vi "BuildConstructor.vi"(7 "PythonConverter_BD in":refnum<class "PyConvBD.lvclass">, 8 "error in":errorcluster, 11 "SubVI in":refnum<class "SubVI.lvclass">) -> (0 "error out":errorcluster, 3 "SubVI out":refnum<class "SubVI.lvclass">, 4 "constructor":string, 5 "PythonConverter_BD out":refnum<class "PyConvBD.lvclass">)   [LabVIEW 2014, in "Raspberry Pi Compatible Compiler for LabVIEW.lvlib" / "SubVI.lvclass"]
uses:
  SubVI.lvclass
  Python/PythonConverter_BD/PyConvBD.lvclass
  SubVI.lvclass/SubVI.ctl
  Node/Node.lvclass
  Python/Parsing/Python Functions.lvlib
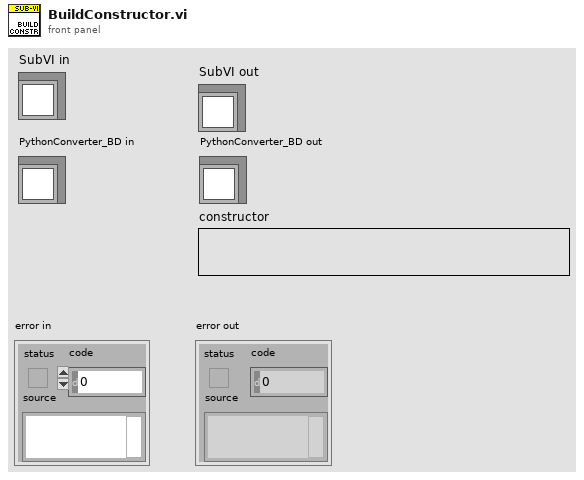
[diagram p1: front panel]
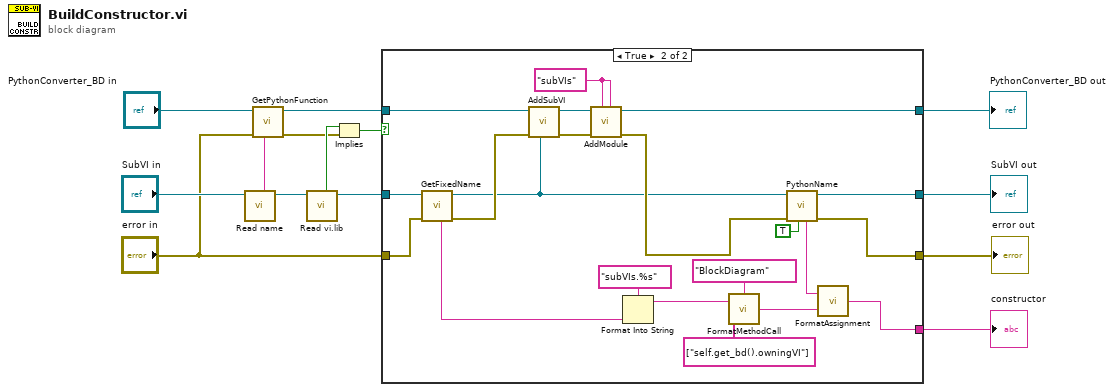
[diagram p0: block diagram]
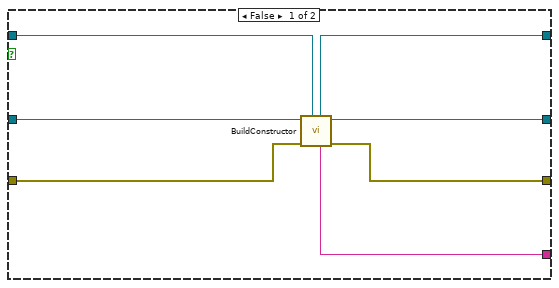
[diagram p2: hidden frame]
diagram:
  n1 = call-dynamic "Read name.vi"("SubVI in"="SubVI in") -> ("SubVI out"=w5:refnum<class "SubVI.lvclass">, "name"=w8:string)  [unwired: 7 in]
  n2 = call "GetPythonFunction.vi"("function name"=w8, "error in"="error in", "PythonConverter_BD in"="PythonConverter_BD in") -> ("error out"=w2:errorcluster, "PythonConverter_BD out"=w9:refnum<class "PyConvBD.lvclass">)  [unwired: 4 in, 1 out]
  n3 = call "Read vi.lib.vi"("SubVI in"=w5) -> ("SubVI out"=w4:refnum<class "SubVI.lvclass">, "vi.lib"=w6:bool)  [unwired: 7 in]
  n4 = Implies(1:w2, 2:w6) -> (0:w7:bool)
  n5 = case shown="True" w7 {
    tunnel: [w15 w37] -> w14
    tunnel: [w21 w38] -> w13
    tunnel: [w20 w34] -> w12
    tunnel: [w19 w32] -> w11
    tunnel: w9 -> [w18 w26]
    tunnel: w4 -> [w17 w29]
    tunnel: "error in" -> [w16 w28]
    frame False {
      n6 = call-parent "BuildConstructor.vi"("PythonConverter_BD in"=w18, "error in"=w16, "Node in"=w17) -> ("error out"=w15:errorcluster, "Node out"=w21:refnum<class "SubVI.lvclass">, "constructor"=w20:string, "PythonConverter_BD out"=w19:refnum<class "PyConvBD.lvclass">)  [unwired: 5 in]
    }
    frame True {
      w30 = "subVIs" ("python module")
      n7 = call-dynamic "GetFixedName.vi"("error in"=w28, "SubVI in"=w29) -> ("error out"=w23:errorcluster, "SubVI out"=w22:refnum<class "SubVI.lvclass">, "fixed name"=w27:string)  [unwired: 5 in]
      n8 = call "AddSubVI.vi"("SubVI"=w22, "error in"=w23, "PythonConverter_BD in"=w26) -> ("error out"=w24:errorcluster, "PythonConverter_BD out"=w25:refnum<class "PyConvBD.lvclass">)  [unwired: 5 in]
      n9 = call "AddModule.vi"("python module name"=w30, "python module"=w30, "error in"=w24, "PythonConverter_BD in"=w25) -> ("error out"=w31:errorcluster, "PythonConverter_BD out"=w32:refnum<class "PyConvBD.lvclass">)  [unwired: 4 in]
      n10 = Format Into String(format string="subVIs.%s", w27) -> (resulting string=w35:string)  [unwired: 2 in, 1 out]
      n11 = call "FormatMethodCall.vi"("method"="BlockDiagram", "parameters"=string[] ["self.get_bd().owningVI"], "object"=w35) -> ("python object"=w39:string)
      n12 = call-dynamic "PythonName.vi"("add self"=TRUE, "error in"=w31, "Node in"=w22) -> ("error out"=w37:errorcluster, "Node out"=w38:refnum<class "SubVI.lvclass">, "name"=w40:string)  [unwired: 5 in, 1 out]
      n13 = call "FormatAssignment.vi"("value"=w39, "name"=w40) -> ("python assignment"=w34:string)
    }
  }
  "error out" <- w14
  "SubVI out" <- w13
  "constructor" <- w12
  "PythonConverter_BD out" <- w11
